vi "7L12-qe_te_0.vi"(6 "err in":errorcluster, 8 "Cc":dbl=20.0, 9 "T":dbl=0.15, 10 "Pu":dbl, 11 "Qa":dbl) -> (2 "Te (en mois)":dbl, 3 "Qe":dbl, 4 "error out":errorcluster caption="err out")   [LabVIEW 2010, in "lv_07.lvlib"]
doc: "Application des formules de Wilson\nCe Vi calcule la quantité économique (Qe) et la période économique (Te) de réapprovisionnement à partir des données de la pièce (Qa,Pu) et de l'entreprise (T=0,15 par défaut,Cc=15 par défaut)"
uses:
  lv_07.lvlib
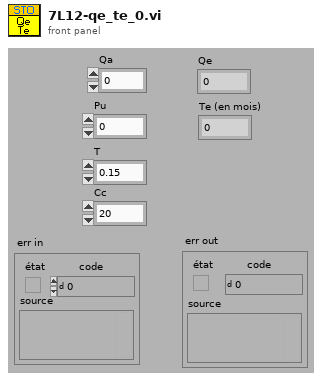
[diagram p1: front panel]
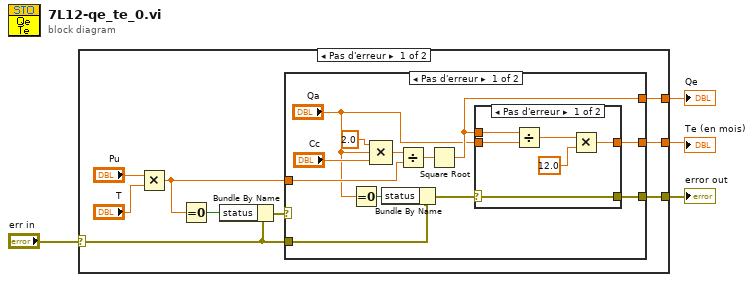
[diagram p0: block diagram]
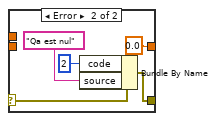
[diagram p2: hidden frame]
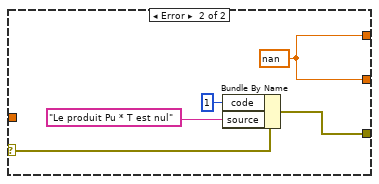
[diagram p3: hidden frame]
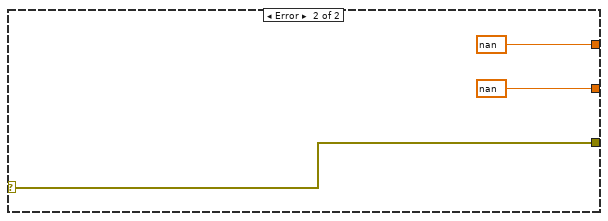
[diagram p4: hidden frame]
diagram:
  n1 = case shown="Pas d'erreur" "err in" {
    selector: "err in" -> [w5 w44]
    tunnel: [w8 w44] -> w4
    tunnel: [w7 nan] -> w3
    tunnel: [w6 nan] -> w2
    frame No Error {
      n2 = Multiply(x="Pu", y="T") -> (x*y=w10:dbl)
      n3 = Equal To 0?(x=w10) -> (x = 0?=w11:bool)
      n4 = Bundle By Name(cluster=w5, "status"=w11) -> (w9:errorcluster)
      n5 = case shown="Pas d'erreur" w9 {
        selector: w9 -> [_ w41]
        tunnel: w10 -> [w21 _]
        tunnel: [w15 w39] -> w8
        tunnel: [w20 w38] -> w7
        tunnel: [w19 w38] -> w6
        tunnel: w5 -> [w14 _]
        frame No Error {
          n6 = Equal To 0?(x="Qa") -> (x = 0?=w17:bool)
          n7 = Compound Arithmetic op=MULTIPLY(2.0, "Qa", "Cc") -> (w24:dbl)
          n8 = Bundle By Name(cluster=w14, "status"=w17) -> (w16:errorcluster)
          n9 = Divide(x=w24, y=w21) -> (x/y=w25:dbl)
          n10 = Square Root(x=w25) -> (sqrt(x)=w20:dbl)
          n11 = case shown="Pas d'erreur" w16 {
            selector: w16 -> [w26 w35]
            tunnel: w20 -> [w29 _]
            tunnel: [w28 0.0] -> w19
            tunnel: "Qa" -> [w27 _]
            tunnel: [w26 w34] -> w15
            frame No Error {
              n12 = Divide(x=w29, y=w27) -> (x/y=w30:dbl)
              n13 = Multiply(x=w30, y=12.0) -> (x*y=w28:dbl)
            }
            frame Error {
              n14 = Bundle By Name(cluster=w35, "code"=2, "source"="Qa est nul") -> (w34:errorcluster)
            }
          }
        }
        frame Error {
          w38 = nan
          n15 = Bundle By Name(cluster=w41, "code"=1, "source"="Le produit Pu * T est nul") -> (w39:errorcluster)
        }
      }
    }
    frame Error {
    }
  }
  "error out" <- w4
  "Qe" <- w3
  "Te (en mois)" <- w2
